vi "Store Waveform to Reference Channel.vi"(8 "error in (no error)":errorcluster, 9 "Reference Channel (5: Reference 1)":u16(ring)=5 items=["Reference 1"=5, "Reference 2"=6, "Reference 3"=7, "Reference 4"=8], 10 "Source Channel (0: Channel 1)":u16(ring) items=["Channel 1", "Channel 2", "Channel 3", "Channel 4", "Math", "Reference 1", "Reference 2", "Reference 3", "Reference 4"], 11 "VISA resource name":refnum<visa-resource-name>) -> (0 "error out":errorcluster, 3 "VISA resource name out":refnum<visa-resource-name>)   [LabVIEW 2009, in "Tektronix DPO MSO 2000 4000 Series.lvlib"]
doc: "Stores a waveform to a reference channel."
uses:
  <instrlib>/Tektronix DPO MSO 2000 4000 Series/Tektronix DPO MSO 2000 4000 Series.lvlib
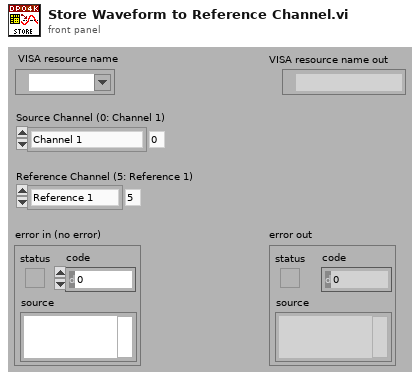
[diagram p1: front panel]
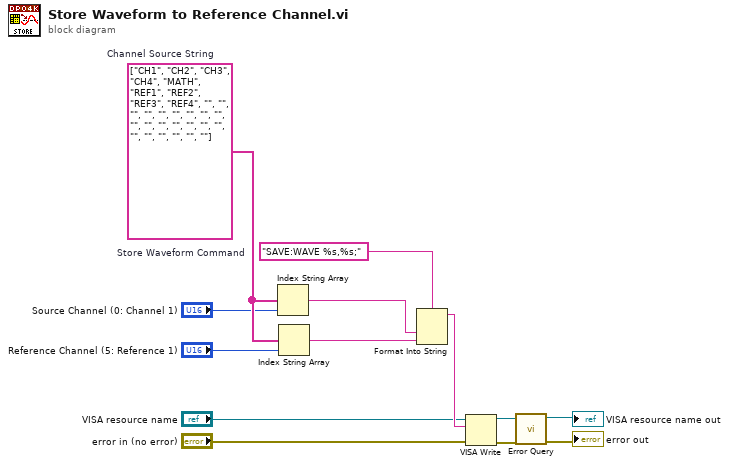
[diagram p0: block diagram]
diagram:
  w12 = "SAVE:WAVE %s,%s;"  # Store Waveform Command
  w7 = string[] ["CH1", "CH2", "CH3", "CH4", "MATH", "REF1", "REF2", "REF3", "REF4", "", "", "", "", "", "", "", "", "", "", "", "", "", "", "", "", "", "", "", "", "", ""]  # Channel Source String
  n1 = Index String Array(1:"Source Channel (0: Channel 1)", 2:w7) -> (0:w11:string)  [unwired: 1 in]
  n2 = Index String Array(1:"Reference Channel (5: Reference 1)", 2:w7) -> (0:w10:string)  [unwired: 1 in]
  n3 = Format Into String(format string=w12, w11, w10) -> (resulting string=w5:string)  [unwired: 2 in, 1 out]
  n4 = VISA Write(VISA resource name="VISA resource name", write buffer=w5, error in (no error)="error in (no error)") -> (VISA resource name out=w2:refnum<visa-resource-name>, error out=w1:errorcluster)  [unwired: 1 out]
  n5 = call <instrlib>:"Error Query.vi"("error in (no error)"=w1, "VISA resource name"=w2) -> ("error out"=→"error out":errorcluster, "VISA resource name out"=→"VISA resource name out":refnum<visa-resource-name>)  [unwired: 6 in, 2 out]
